vi "Get Self Alias.vi"(10 "Addresses DVR":refnum<data-value>) -> (0 "error out":errorcluster, 2 "Self Alias":string)   [LabVIEW 2021, in "jettl.lvlib" / "Addresses.lvlib"]
uses:
  Addresses.lvlib
  Addresses/Addresses.lvclass
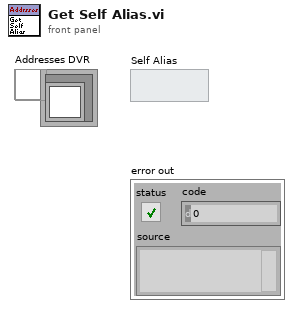
[diagram p1: front panel]
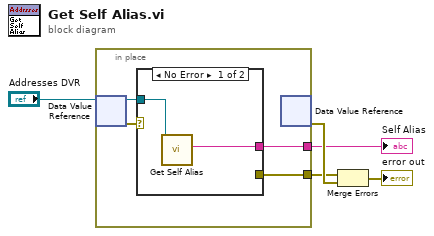
[diagram p0: block diagram]
diagram:
  n1 = in-place {
    in-place-border: [w9] -> w3
    in-place-border: [w8] -> w1
    n2 = in-place-dvr #1("Addresses DVR") -> (w6:refnum<class "Addresses.lvclass">, w7:errorcluster)
    n3 = case shown="No Error" w7 {
      selector: w7 -> [_ w12]
      tunnel: w6 -> [w11 _]
      tunnel: [_ w12] -> w9
      tunnel: [w10 _] -> w8
      frame No Error {
        n4 = call "Get Self Alias.vi"("Addresses in"=w11) -> ("Self Alias"=w10:string)  [unwired: 10 in]
      }
      frame Error {
      }
    }
    n5 = in-place-dvr #1() -> (w4:errorcluster)  [unwired: 1 in, 1 out]
  }
  "Self Alias" <- w1
  n6 = Merge Errors(w3, w4) -> (→"error out":errorcluster)
